vi "Write Transformation matrix.vi"(8 "error in (no error)":errorcluster, 10 "Transformation matrix":dbl[][](array[numeric]), 11 "Transform in":refnum<class "Transform.lvclass">) -> (0 "error out":errorcluster, 3 "Transform out":refnum<class "Transform.lvclass">)   [LabVIEW 2013, in "HardwareCharacterization.lvlib" / "Transform.lvclass"]
uses:
  Transform.lvclass
  Transform.lvclass/Transform.ctl
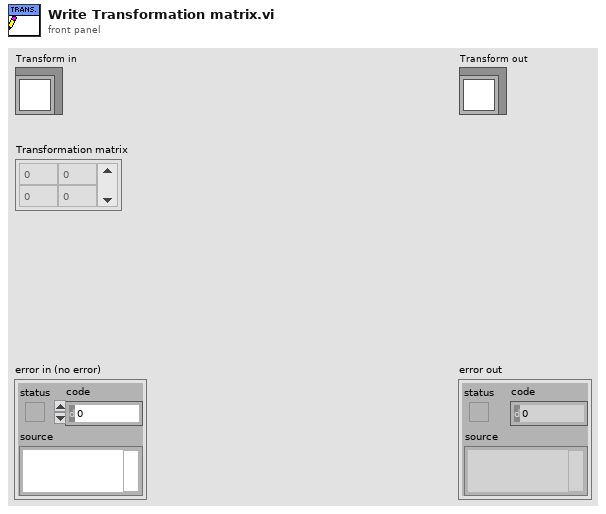
[diagram p1: front panel]
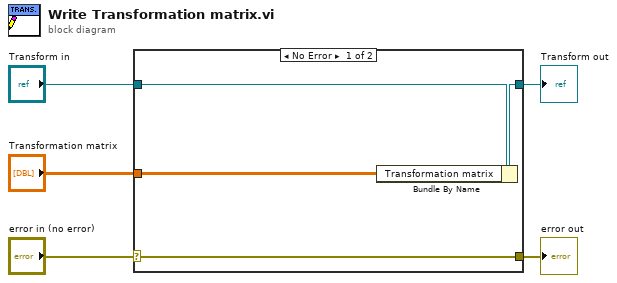
[diagram p0: block diagram]
diagram:
  n1 = case shown="No Error" "error in (no error)" {
    selector: "error in (no error)" -> [w9 w10]
    tunnel: [w9 w10] -> w4
    tunnel: [w7 w11] -> w2
    tunnel: "Transform in" -> [w8 w11]
    tunnel: "Transformation matrix" -> [w6 _]
    frame No Error {
      n2 = Bundle By Name(cluster=w8, "Transformation matrix"=w6) -> (w7:refnum<class "Transform.lvclass">)
    }
    frame Error {
    }
  }
  "error out" <- w4
  "Transform out" <- w2
